vi "I2C Controller Module.vi"(11 "error in (no error)":errorcluster) -> (15 "error out":errorcluster)   [LabVIEW 2020, in "I2C Controller Lib.lvlib"]
uses:
  I2C Controller Lib.lvlib
  TypeDef/Transmission Data.ctl
  TypeDef/DVR Cluster.ctl
  Class/Transmission Mode/Parent/TX Speed.lvclass
  Class/Addressing Mode/Parent/Addressing Mode.lvclass
  Class/Devices/Parent/Devices.lvclass
  TypeDef/Path Cluster.ctl
  TypeDef/Queue Operation Mode.ctl
  TypeDef/User LV2 Mode Select.ctl
  <vilib>/Utility/config.llb/Read Key (String).vi
  Class/Transmission Mode/Child/Low Speed/SubVI/SubPanel.vi
  <vilib>/Utility/config.llb/NI_LVConfig.lvlib
  Class/Transmission Mode/Child/Low Speed/Low Speed.lvclass
panel:
  in  "Clear?":bool
  in  "Configure?":bool
  out "Warning":string caption="Warning:"
  in  "TX.Data":T1=[10, 188, 218, 14, 47, 69, 255, 107, 7, 92, 64] caption="Transmission Data" format="%.0x"
  out "RX.Data":u8[](array[numeric]) caption="Read Bytes" format="%.0x"
  out "Acknoledge?":bool caption="ACK / NACK"
  in  "Speed Mode":string(combo)="Select Device"
  in  "Transmit Data?":bool caption="Start Transmission"
  in  "Add Device?":bool caption="Add DEvice?"
  in  "Oper. Mode":string(combo)="Select Operation" caption="Operation Mode"
  in  "Address Mode":enum32{"7-bit", "10-Bit"}(radio) caption="Addressing Mode"
  in  "Log.Open?":bool
  in  "Target Address":u16=26 max=128 step=1 format="%.0x"
  in  "Device Type":string(combo)="Select Device Type"
  in  "Voltage":dbl=1.8 caption="Voltage (V)" min=1.8 max=5.0 step=1.0 format="%.2g"
  out "Digital Waveform Graph":digitaldata[](graph) caption="Graph"
  # "I2C Controller Module"
  # "Controller"
  # "Target"
  # "Transmission Parameters"
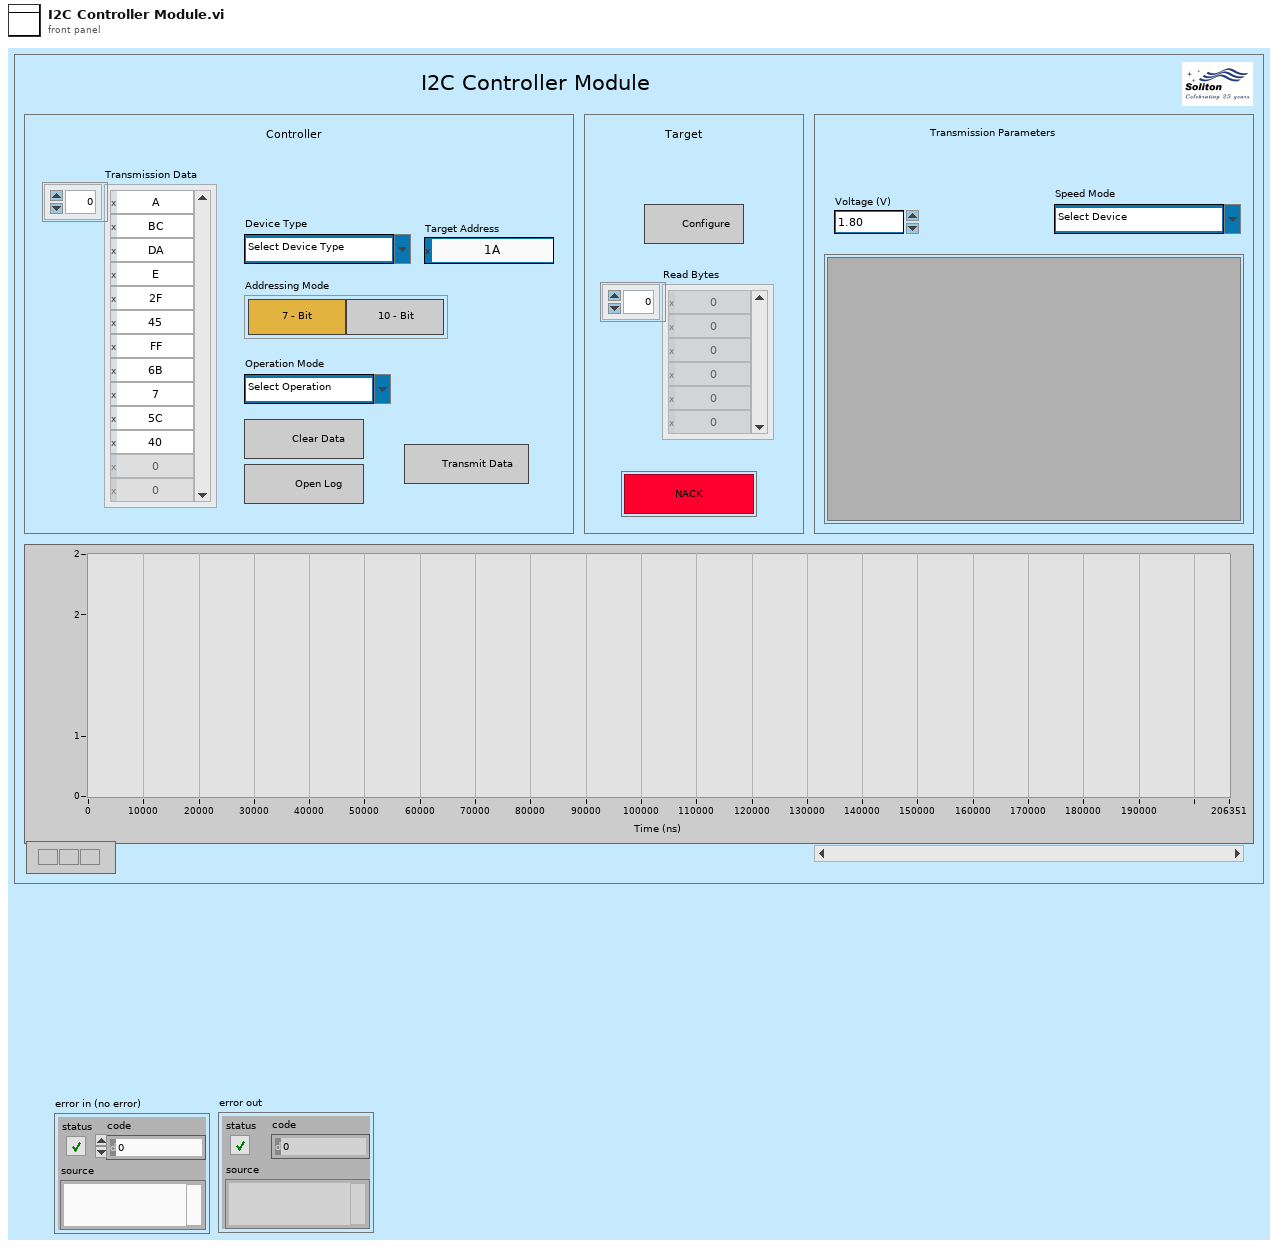
[diagram p1: front panel]
types:
  T1 = typedef "I2C Controller Lib.lvlib/Transmission Data.ctl" = u8[]
  T2 = typedef "I2C Controller Lib.lvlib/User LV2 Mode Select.ctl" = enum16{"Create", "Delete", "Stop"}
  T3 = typedef "I2C Controller Lib.lvlib/Queue Operation Mode.ctl" = enum16{"Create Q", "Enqueue", "Enqueue N", "Enstack", "Dequeue", "Flush Q", "Close Q"}
  T4 = typedef "I2C Controller Lib.lvlib/DVR Cluster.ctl" = cluster{"TX. Mode":refnum<data-value>, "Addr. Mode":refnum<data-value>, "Devices":refnum<data-value>}
  T5 = typedef "I2C Controller Lib.lvlib/Path Cluster.ctl" = cluster{"Config File":path, "TX.Mode":path, "Devices":path, "Addr. Mode":path}
  T6 = cluster{"Enable/Disable":string, "Warning":string, "Oper. Mode":string, "Speed Mode":string, "Address Mode":enum32{"7-bit", "10-Bit"}, "TX.Data":T1, "Device Type":string, "DVR":T4, "Path":T5, "Flags":cluster{"Device Type":bool, "Speed Mode":bool, "Target Address":bool, "Oper. Mode":bool}, "RX.Data":u8[], "Acknoledge?":bool, "Graph Wave":digitaldata[]}
  T7 = typedef "NI_LVConfig.lvlib/Config Data RefNum.ctl" = refnum<k1>
  T8 = enum8{"Enabled", "Disabled", "Disabled and Grayed Out"}
  T9 = cluster{"Device Type":bool, "Speed Mode":bool, "Target Address":bool, "Oper. Mode":bool}
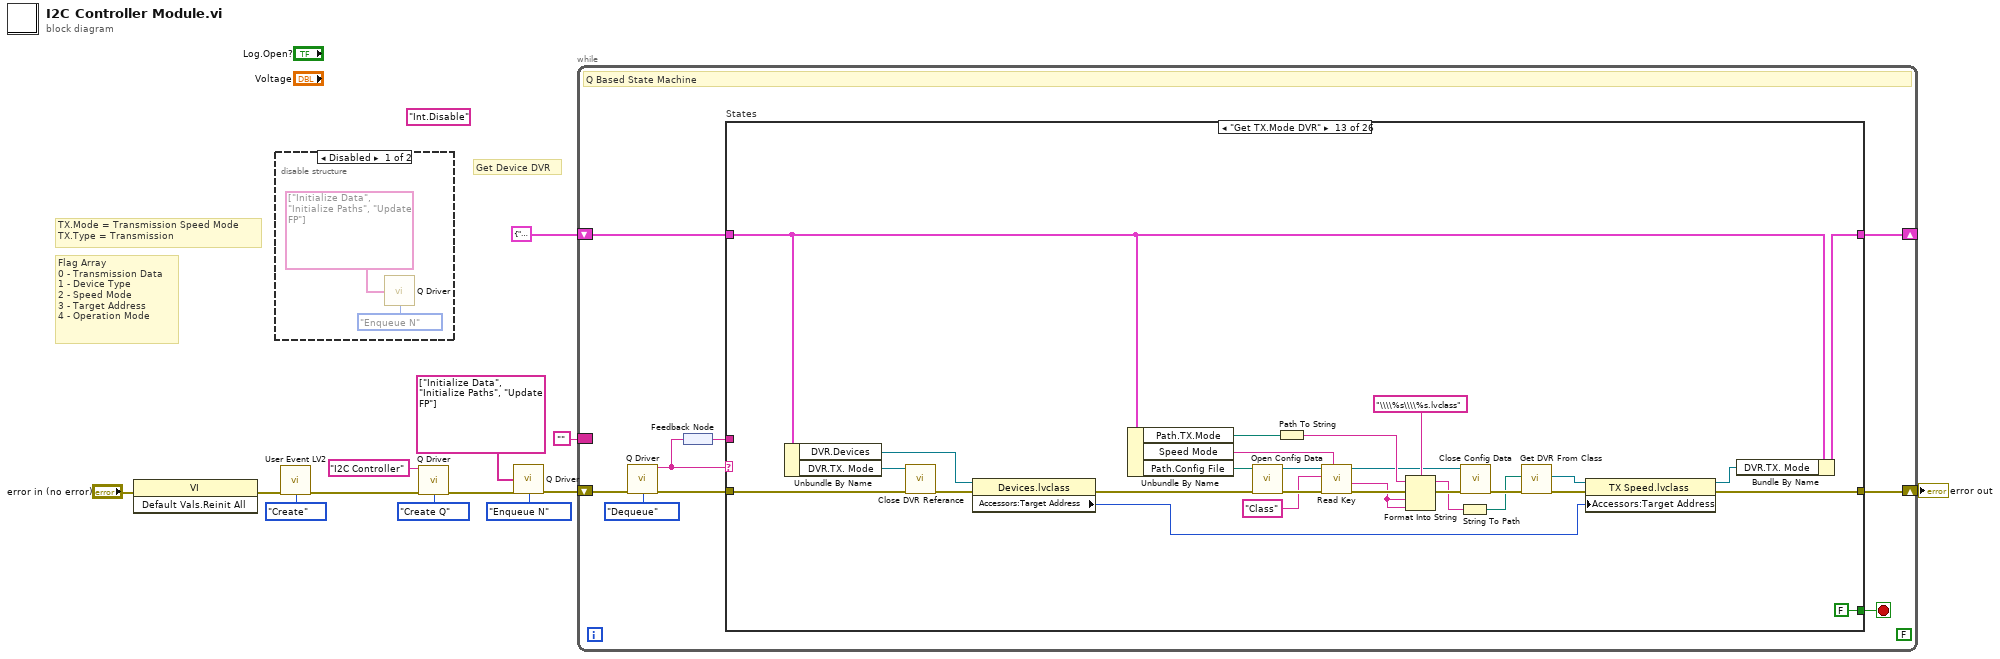
[diagram p0: block diagram]
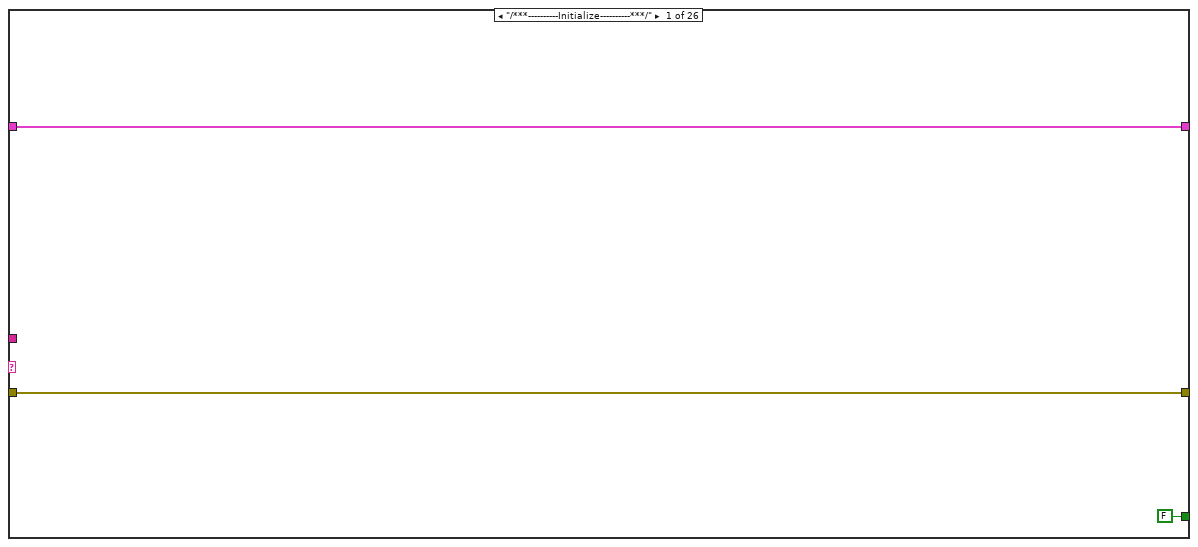
[diagram p3: hidden frame]
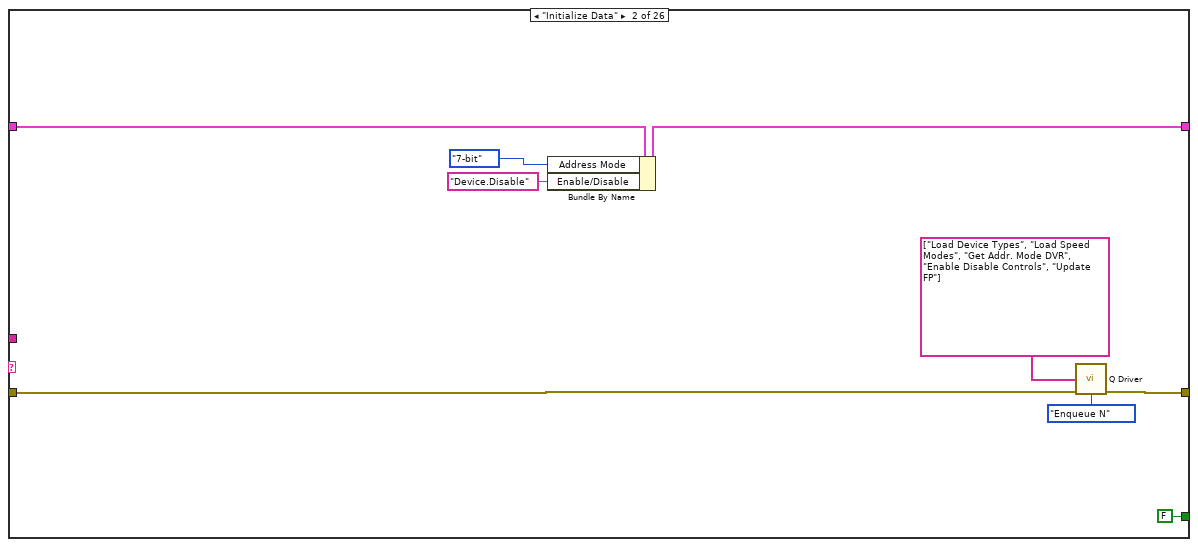
[diagram p4: hidden frame]
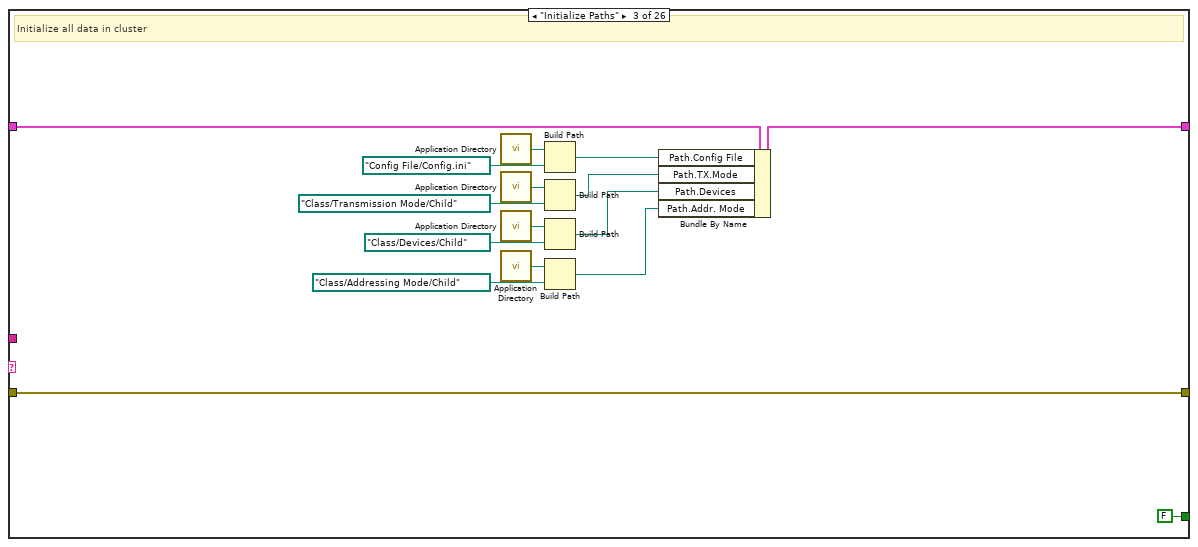
[diagram p5: hidden frame]
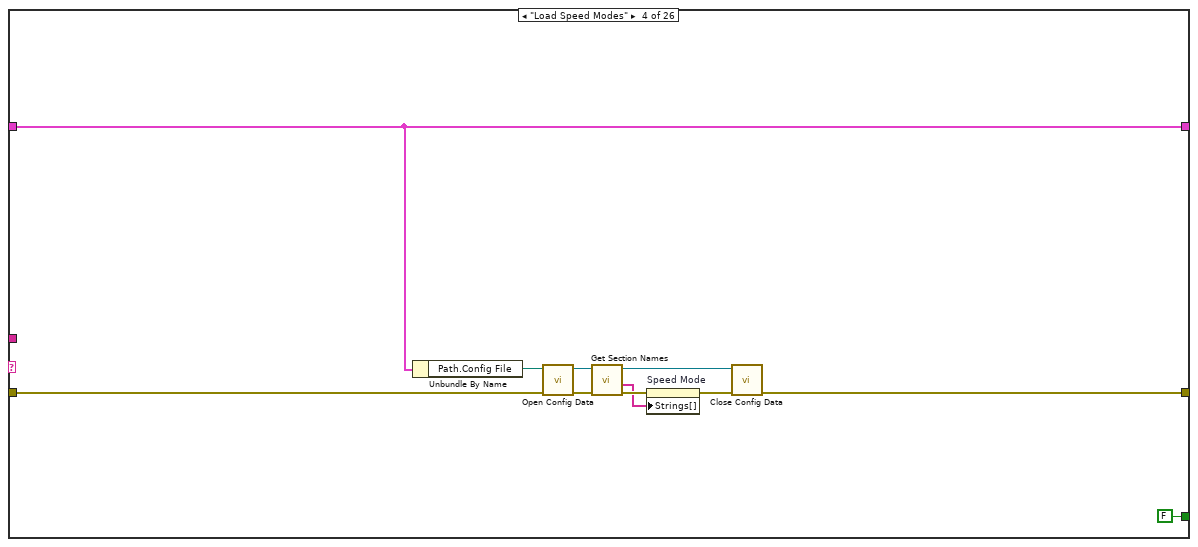
[diagram p6: hidden frame]
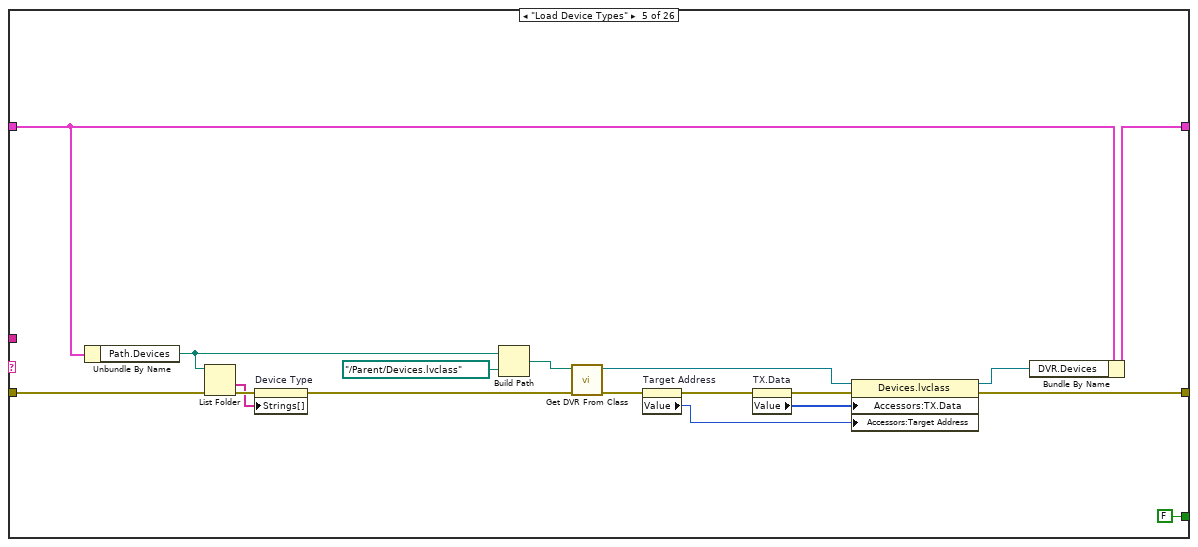
[diagram p7: hidden frame]
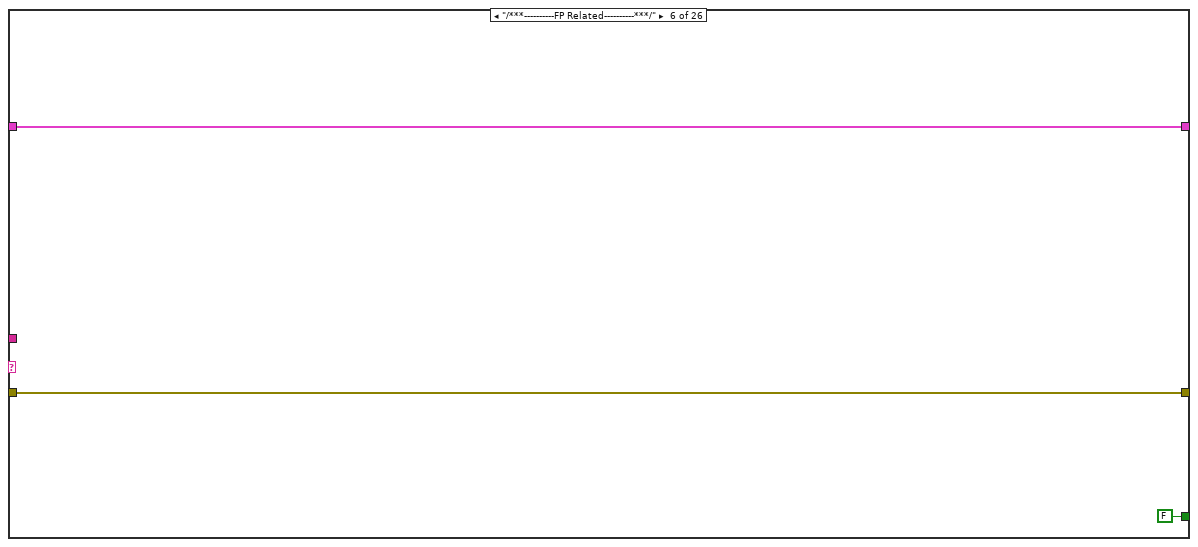
[diagram p8: hidden frame]
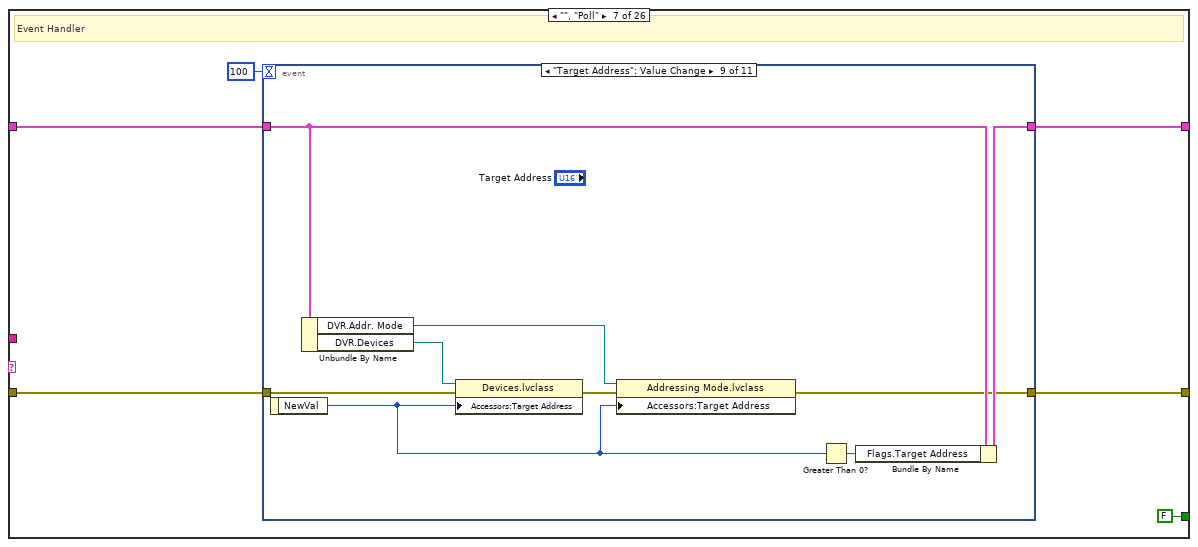
[diagram p9: hidden frame]
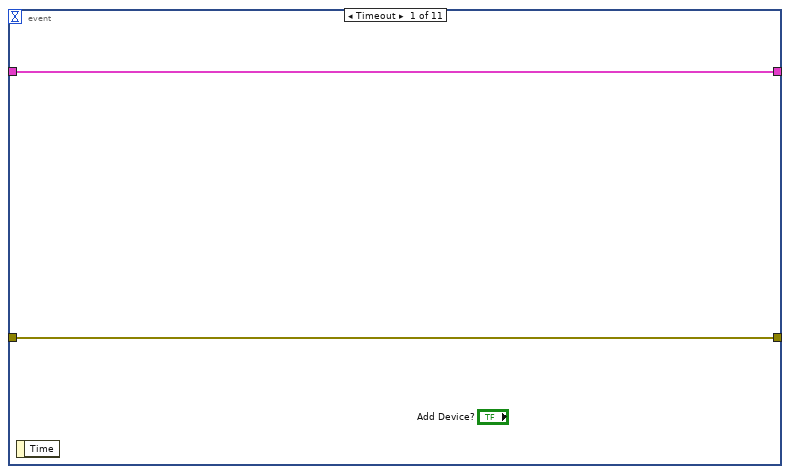
[diagram p10: hidden frame]
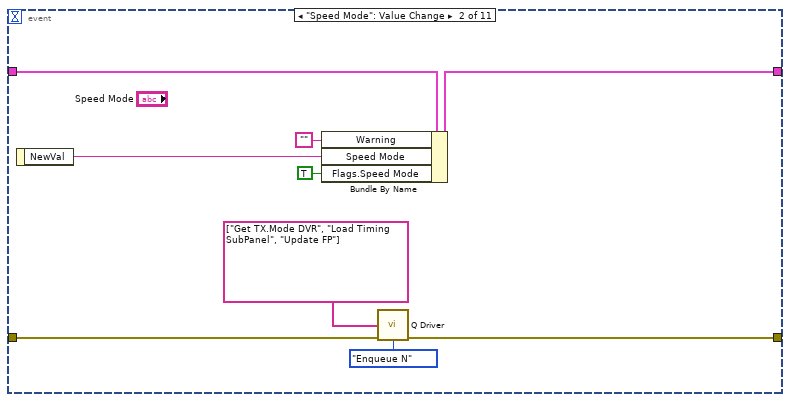
[diagram p11: hidden frame]
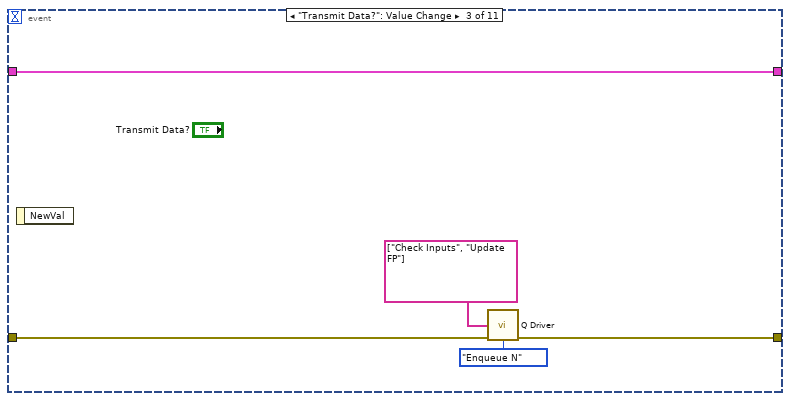
[diagram p12: hidden frame]
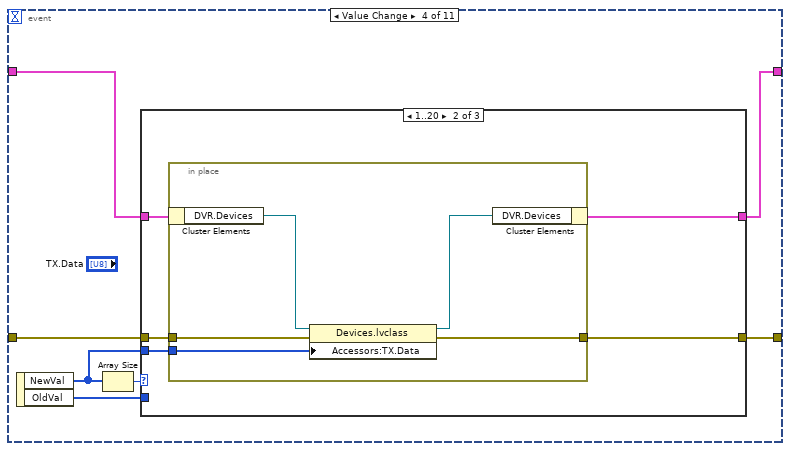
[diagram p13: hidden frame]
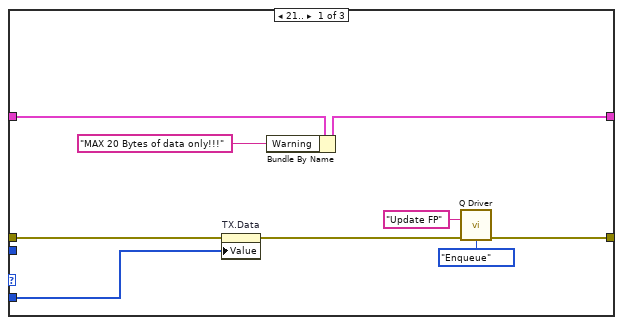
[diagram p14: hidden frame]
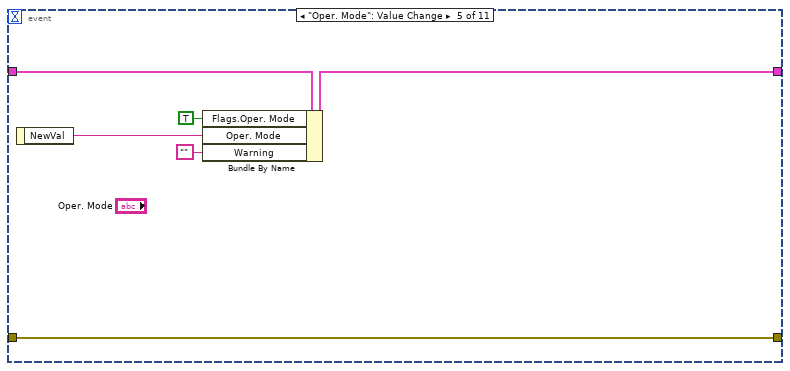
[diagram p16: hidden frame]
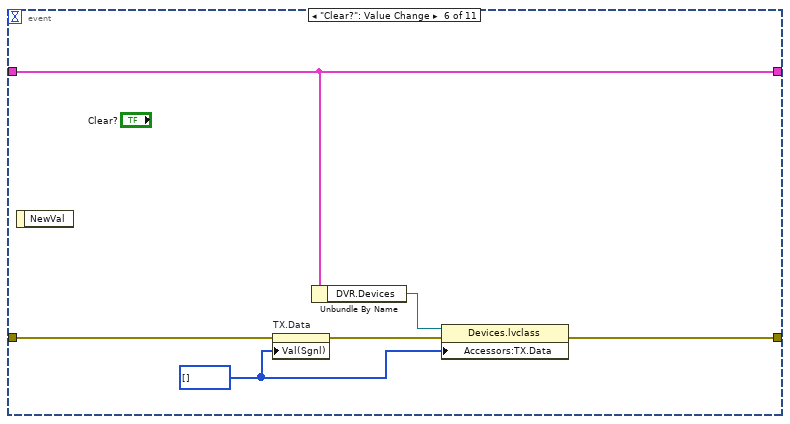
[diagram p17: hidden frame]
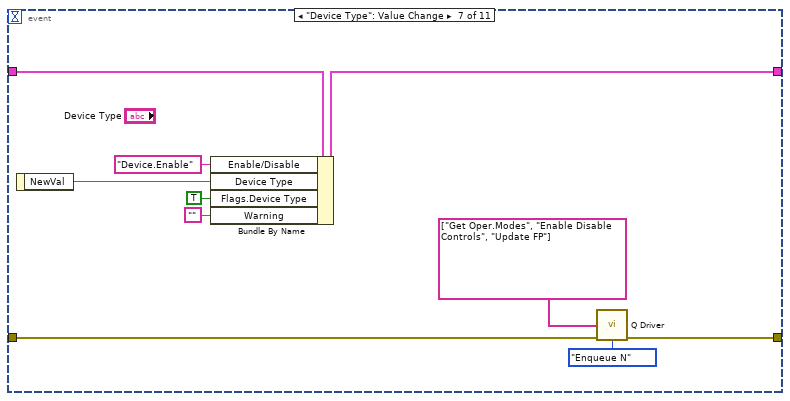
[diagram p18: hidden frame]
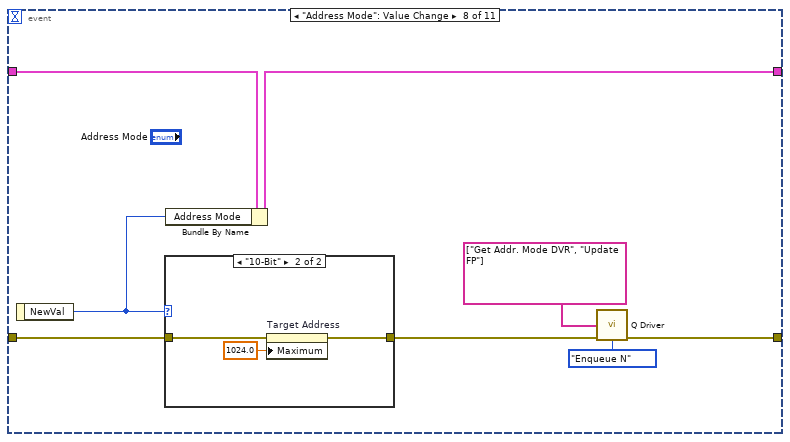
[diagram p19: hidden frame]
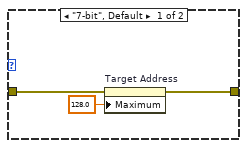
[diagram p20: hidden frame]
diagram:
  (unwired) "Int.Disable" ("Enable/Disable")
  # "Get Device DVR"
  # "Flag Array\n0 - Transmission Data\n1 - Device Type\n2 - Speed Mode\n3 - Target Address\n4 - Operation Mode"
  # "TX.Mode = Transmission Speed Mode\nTX.Type = Transmission"
  n1 = invoke class="VI" method="Default Vals.Reinit All"(error in="error in (no error)") -> (error out=w2:errorcluster)  [unwired: 2 in, 2 out]
  n2 = disable-structure shown="Disabled" {
    frame Disabled {
      n3 = call "Q Driver.vi"("States s[]"=string[] ["Initialize Data", "Initialize Paths", "Update FP"], "Q Operation"=Queue_Operation_Mode."Enqueue N") -> ()  [unwired: 12 in, 2 out]
    }
    frame Enabled {
    }
  }
  n4 = call "User Event LV2.vi"("error in (no error)"=w2, "LV2 Mode"=User_LV2_Mode_Select."Create") -> ("error out"=w1:errorcluster)  [unwired: 12 in, 1 out]
  n5 = call "Q Driver.vi"("Q Name"="I2C Controller", "error in (no error)"=w1, "Q Operation"=Queue_Operation_Mode."Create Q") -> ("error out"=w12:errorcluster)  [unwired: 11 in, 1 out]
  n6 = call "Q Driver.vi"("States s[]"=string[] ["Initialize Data", "Initialize Paths", "Update FP"], "error in (no error)"=w12, "Q Operation"=Queue_Operation_Mode."Enqueue N") -> ("error out"=w11:errorcluster)  [unwired: 11 in, 1 out]
  n7 = while {
    shift-right: [w21] -> _
    shift-left: T6 {"Enable/Disable"="", "Warning"="", "Oper. Mode"="", "Speed Mode"="", "Address Mode"=enum."7-bit", "TX.Data"=[], "Device Type"="", "DVR"={"TX. Mode"=refnum, "Addr. Mode"=refnum, "Devices"=refnum}, "Path"={"Config File"=path "", "TX.Mode"=path "", "Devices"=path "", "Addr. Mode"=path ""}, "Flags"={"Device Type"=FALSE, "Speed Mode"=FALSE, "Target Address"=TRUE, "Oper. Mode"=FALSE}, "RX.Data"=[], "Acknoledge?"=FALSE, "Graph Wave"=[]} -> [w20]
    shift-right: [w22] -> w8
    shift-left: w11 -> [w24]
    border: "" -> [_]
    stop <- w19 stop-if-true
    (unwired) FALSE
    # "Q Based State Machine"
    n8 = call "Q Driver.vi"("error in (no error)"=w24, "Q Operation"=Queue_Operation_Mode."Dequeue") -> ("State Out"=w17:string, "error out"=w23:errorcluster)  [unwired: 12 in]
    n9 = feedback-in #1(w17) -> ()
    n10 = feedback #1() -> (w16:string)
    n11 = case "States" shown="\"Get TX.Mode DVR\"" w17 {
      selector: w17 -> [_ _ _ _ _ _ _ _ _ _ _ _ _ _ _ _ _ _ _ _ _ _ _ w468 _ _]
      tunnel: w23 -> [w27 w31 w40 w62 w80 w84 w90 w207 w227 w230 w236 w250 w289 w309 w320 w326 w330 w345 w373 w426 w443 w446 w449 w470 w491 w496]
      tunnel: [w27 w30 w40 w56 w69 w84 w89 w208 w227 w230 w238 w253 w282 w309 w319 w325 w330 w337 w371 w415 w441 w446 w448 w469 w491 w494] -> w22
      tunnel: [w26 w35 w50 w54 w74 w83 w87 w206 w225 w229 w237 w254 w291 w308 w321 w324 w329 w340 w374 w413 w429 w445 w460 w481 w490 w498] -> w21
      tunnel: w20 -> [w26 w36 w51 w54 w79 w83 w86 w206 w225 w229 w244 w252 w288 w308 w321 w324 w329 w340 w376 w423 w442 w445 w460 w481 w490 w498]
      tunnel: [FALSE FALSE FALSE FALSE FALSE FALSE FALSE FALSE FALSE FALSE FALSE FALSE FALSE FALSE FALSE FALSE FALSE FALSE FALSE FALSE FALSE FALSE FALSE FALSE FALSE TRUE] -> w19
      tunnel: w16 -> [_ _ _ _ _ _ _ _ _ _ _ _ _ _ _ _ _ _ _ _ _ _ w447 _ _ _]
      frame "/***----------Initialize----------***/" {
      }
      frame "Initialize Data" {
        n12 = Bundle By Name(cluster=w36, "Address Mode"=enum32{"7-bit", "10-Bit"}."7-bit", "Enable/Disable"="Device.Disable") -> (w35:T6)
        n13 = call "Q Driver.vi"("States s[]"=string[] ["Load Device Types", "Load Speed Modes", "Get Addr. Mode DVR", "Enable Disable Controls", "Update FP"], "error in (no error)"=w31, "Q Operation"=Queue_Operation_Mode."Enqueue N") -> ("error out"=w30:errorcluster)  [unwired: 11 in, 1 out]
      }
      frame "Initialize Paths" {
        # "Initialize all data in cluster"
        n14 = call <vilib>:"Application Directory.vi"() -> ("Application Directory"=w49:path)
        n15 = call <vilib>:"Application Directory.vi"() -> ("Application Directory"=w45:path)
        n16 = call <vilib>:"Application Directory.vi"() -> ("Application Directory"=w43:path)
        n17 = call <vilib>:"Application Directory.vi"() -> ("Application Directory"=w39:path)
        n18 = Build Path(base path=w49, name or relative path=path "Config File/Config.ini" ("Config.ini")) -> (appended path=w47:path)
        n19 = Build Path(base path=w45, name or relative path=path "Class/Transmission Mode/Child" ("Config.ini")) -> (appended path=w44:path)
        n20 = Build Path(base path=w43, name or relative path=path "Class/Devices/Child" ("Config.ini")) -> (appended path=w41:path)
        n21 = Build Path(base path=w39, name or relative path=path "Class/Addressing Mode/Child" ("Config.ini")) -> (appended path=w37:path)
        n22 = Bundle By Name(cluster=w51, "Path.Config File"=w47, "Path.TX.Mode"=w44, "Path.Devices"=w41, "Path.Addr. Mode"=w37) -> (w50:T6)
      }
      frame "Load Speed Modes" {
        n23 = Unbundle By Name(w54) -> ("Path.Config File"=w53:path)
        n24 = call <vilib>:"Open Config Data.vi"("error in (no error)"=w62, "configuration file path"=w53) -> ("error out"=w61:errorcluster, "refnum"=w60:T7)  [unwired: 7 in, 1 out]
        n25 = call <vilib>:"Get Section Names.vi"("error in (no error)"=w61, "refnum"=w60) -> ("error out"=w59:errorcluster, "section names"=w58:string[], "refnum out"=w55:T7)  [unwired: 7 in]
        n26 = property on="Speed Mode" class="CmbBox"(error in=w59, "Strings[]"=w58) -> (error out=w57:errorcluster)  [unwired: 1 in, 1 out]
        n27 = call <vilib>:"Close Config Data.vi"("error in (no error)"=w57, "refnum"=w55) -> ("error out"=w56:errorcluster)  [unwired: 8 in, 1 out]
      }
      frame "Load Device Types" {
        n28 = Unbundle By Name(w79) -> ("Path.Devices"=w73:path)
        n29 = List Folder(path=w73, error in=w80) -> (folder names=w77:string[], error out=w78:errorcluster)  [unwired: 2 in, 2 out]
        n30 = property on="Device Type" class="CmbBox"(error in=w78, "Strings[]"=w77) -> (error out=w76:errorcluster)  [unwired: 1 in, 1 out]
        n31 = Build Path(base path=w73, name or relative path=path "../Parent/Devices.lvclass") -> (appended path=w72:path)
        n32 = call "Get DVR From Class.vi"("error in (no error)"=w76, "Path In"=w72) -> ("error out"=w75:errorcluster, "Devices DVR"=w68:refnum<data-value>)  [unwired: 8 in]
        n33 = property on="Target Address" class="DigNum (strict)"(error in=w75) -> (error out=w65:errorcluster, "Value"=w64:u16)  [unwired: 1 in, 1 out]
        n34 = property on="TX.Data" class="Arr (strict)"(error in=w65) -> (error out=w70:errorcluster, "Value"=w67:T1)  [unwired: 1 in, 1 out]
        n35 = property class="Devices.lvclass"(reference=w68, error in=w70, "Accessors:TX.Data"=w67, "Accessors:Target Address"=w64) -> (reference out=w66:refnum<data-value>, error out=w69:errorcluster)
        n36 = Bundle By Name(cluster=w79, "DVR.Devices"=w66) -> (w74:T6)
      }
      frame "/***----------FP Related----------***/" {
      }
      frame "", "Poll" {
        # "Event Handler"
        n37 = event shown="[8] \"Target Address\": Value Change" {
          selector: _ -> [_ _ _ _ _ _ _ _ _ _ _]
          dyn-events: _ -> [_ _ _ _ _ _ _ _ _ _ _]
          timeout: 100 -> [_ _ _ _ _ _ _ _ _ _ _]
          tunnel: w90 -> [w92 w97 w103 w113 w135 w146 w153 w163 w177 w186 w203]
          tunnel: [w92 w96 w102 w112 w135 w143 w152 w160 w172 w185 w202] -> w89
          tunnel: [w91 w100 w106 w107 w139 w144 w148 w158 w179 w183 w201] -> w87
          tunnel: w86 -> [w91 w101 w106 w111 w140 w144 w156 w164 w175 w182 w201]
          event Timeout {
            n38 = event-data() -> ()  [unwired: 1 in, 1 out]
          }
          event "Speed Mode": Value Change {
            n39 = event-data() -> ("NewVal"=w99:string)  [unwired: 1 in]
            n40 = Bundle By Name(cluster=w101, "Warning"="", "Speed Mode"=w99, "Flags.Speed Mode"=TRUE) -> (w100:T6)
            n41 = call "Q Driver.vi"("States s[]"=string[] ["Get TX.Mode DVR", "Load Timing SubPanel", "Update FP"], "error in (no error)"=w97, "Q Operation"=Queue_Operation_Mode."Enqueue N") -> ("error out"=w96:errorcluster)  [unwired: 11 in, 1 out]
          }
          event "Transmit Data?": Value Change {
            n42 = event-data() -> ()  [unwired: 1 in, 1 out]
            n43 = call "Q Driver.vi"("States s[]"=string[] ["Check Inputs", "Update FP"], "error in (no error)"=w103, "Q Operation"=Queue_Operation_Mode."Enqueue N") -> ("error out"=w102:errorcluster)  [unwired: 11 in, 1 out]
          }
          event Value Change {
            n44 = event-data() -> ("NewVal"=w110:T1, "OldVal"=w108:T1)  [unwired: 1 in]
            n45 = Array Size(array=w110) -> (size(s)=w109:i32)
            n46 = case shown="1..20" w109 {
              tunnel: w113 -> [w121 w127 w133]
              tunnel: [w119 w123 w134] -> w107
              tunnel: [w115 w126 w133] -> w112
              tunnel: w111 -> [w122 w124 w134]
              tunnel: w110 -> [_ w125 _]
              tunnel: w108 -> [w120 _ _]
              frame 21.. {
                n47 = property on="TX.Data" class="Arr (strict)"(error in=w121, "Value"=w120) -> (error out=w116:errorcluster)  [unwired: 1 in, 1 out]
                n48 = Bundle By Name(cluster=w122, "Warning"="MAX 20 Bytes of data only!!!") -> (w119:T6)
                n49 = call "Q Driver.vi"("State In"="Update FP" ("element"), "error in (no error)"=w116, "Q Operation"=Queue_Operation_Mode."Enqueue") -> ("error out"=w115:errorcluster)  [unwired: 11 in, 1 out]
              }
              frame 1..20 {
                n50 = in-place {
                  in-place-border: w127 -> [w132]
                  in-place-border: [w131] -> w126
                  in-place-border: w125 -> [w130]
                  n51 = in-place-cluster #2(w124) -> ("DVR.Devices"=w129:refnum<data-value>)
                  n52 = property class="Devices.lvclass"(reference=w129, error in=w132, "Accessors:TX.Data"=w130) -> (reference out=w128:refnum<data-value>, error out=w131:errorcluster)
                  n53 = in-place-cluster #2("DVR.Devices"=w128) -> (w123:T6)
                }
              }
              frame 0, Default {
              }
            }
          }
          event "Oper. Mode": Value Change {
            n54 = event-data() -> ("NewVal"=w137:string)  [unwired: 1 in]
            n55 = Bundle By Name(cluster=w140, "Flags.Oper. Mode"=TRUE, "Oper. Mode"=w137, "Warning"="") -> (w139:T6)
          }
          event "Clear?": Value Change {
            w141 = T1 [] ("TX.Data")
            n56 = event-data() -> ()  [unwired: 1 in, 1 out]
            n57 = property on="TX.Data" class="Arr (strict)"(error in=w146, "Val(Sgnl)"=w141) -> (error out=w145:errorcluster)  [unwired: 1 in, 1 out]
            n58 = Unbundle By Name(w144) -> ("DVR.Devices"=w142:refnum<data-value>)
            n59 = property class="Devices.lvclass"(reference=w142, error in=w145, "Accessors:TX.Data"=w141) -> (error out=w143:errorcluster)  [unwired: 1 out]
          }
          event "Device Type": Value Change {
            n60 = event-data() -> ("NewVal"=w155:string)  [unwired: 1 in]
            n61 = Bundle By Name(cluster=w156, "Enable/Disable"="Device.Enable", "Device Type"=w155, "Flags.Device Type"=TRUE, "Warning"="") -> (w148:T6)
            n62 = call "Q Driver.vi"("States s[]"=string[] ["Get Oper.Modes", "Enable Disable Controls", "Update FP"], "error in (no error)"=w153, "Q Operation"=Queue_Operation_Mode."Enqueue N") -> ("error out"=w152:errorcluster)  [unwired: 11 in, 1 out]
          }
          event "Address Mode": Value Change {
            n63 = event-data() -> ("NewVal"=w157:enum32{"7-bit", "10-Bit"})  [unwired: 1 in]
            n64 = case shown="\"10-Bit\"" w157 {
              tunnel: [w165 w169] -> w161
              tunnel: w163 -> [w166 w170]
              frame "7-bit", Default {
                n65 = property on="Target Address" class="DigNum (strict)"(error in=w166, "Maximum"=128.0 ("Data Entry Limits:Maximum")) -> (error out=w165:errorcluster)  [unwired: 1 in, 1 out]
              }
              frame "10-Bit" {
                n66 = property on="Target Address" class="DigNum (strict)"(error in=w170, "Maximum"=1024.0 ("Data Entry Limits:Maximum")) -> (error out=w169:errorcluster)  [unwired: 1 in, 1 out]
              }
            }
            n67 = Bundle By Name(cluster=w164, "Address Mode"=w157) -> (w158:T6)
            n68 = call "Q Driver.vi"("States s[]"=string[] ["Get Addr. Mode DVR", "Update FP"], "error in (no error)"=w161, "Q Operation"=Queue_Operation_Mode."Enqueue N") -> ("error out"=w160:errorcluster)  [unwired: 11 in, 1 out]
          }
          event "Target Address": Value Change {
            n69 = event-data() -> ("NewVal"=w171:u16)  [unwired: 1 in]
            n70 = Unbundle By Name(w175) -> ("DVR.Addr. Mode"=w173:refnum<data-value>, "DVR.Devices"=w174:refnum<data-value>)
            n71 = property class="Devices.lvclass"(reference=w174, error in=w177, "Accessors:Target Address"=w171) -> (error out=w176:errorcluster)  [unwired: 1 out]
            n72 = property class="Addressing Mode.lvclass"(reference=w173, error in=w176, "Accessors:Target Address"=w171) -> (error out=w172:errorcluster)  [unwired: 1 out]
            n73 = Greater Than 0?(x=w171) -> (x > 0?=w178:bool)
            n74 = Bundle By Name(cluster=w175, "Flags.Target Address"=w178) -> (w179:T6)
          }
          event "Configure?": Value Change {
            n75 = event-data() -> ()  [unwired: 1 in, 1 out]
            n76 = Unbundle By Name(w182) -> ("Flags.Device Type"=w184:bool, "Flags.Oper. Mode"=w180:bool)
            n77 = And(x=w184, y=w180) -> (x .and. y?=w181:bool)
            n78 = case shown="True" w181 {
              tunnel: w186 -> [w189 w197]
              tunnel: [w188 w196] -> w185
              tunnel: [w192 w194] -> w183
              tunnel: w182 -> [w193 w194]
              frame False {
                n79 = call "Q Driver.vi"("State In"="Update FP" ("element"), "error in (no error)"=w189, "Q Operation"=Queue_Operation_Mode."Enqueue") -> ("error out"=w188:errorcluster)  [unwired: 11 in, 1 out]
                n80 = Bundle By Name(cluster=w193, "Warning"="Select Device Type and Operation Mode") -> (w192:T6)
              }
              frame True {
                n81 = call "Q Driver.vi"("States s[]"=string[] ["Get Device DVR", "Config RX data", "Update FP"], "error in (no error)"=w197, "Q Operation"=Queue_Operation_Mode."Enqueue N") -> ("error out"=w196:errorcluster)  [unwired: 11 in, 1 out]
              }
            }
          }
          event Panel Close? {
            n82 = event-data() -> ()  [unwired: 1 in, 1 out]
            n83 = call "Q Driver.vi"("State In"="Exit" ("Q Name"), "error in (no error)"=w203, "Q Operation"=Queue_Operation_Mode."Enqueue") -> ("error out"=w202:errorcluster)  [unwired: 11 in, 1 out]
            n84 = event-data("Discard?"=TRUE) -> ()  [unwired: 1 in, 1 out]
          }
        }
      }
      frame "Enable Disable Controls" {
        # "Enable Disable required controls"
        n85 = Unbundle By Name(w206) -> ("Enable/Disable"=w205:string)
        n86 = case shown="\"Device.Disable\"" w205 {
          tunnel: [w210 w212 w216] -> w208
          tunnel: w207 -> [w210 w215 w219]
          frame Default {
          }
          frame "Device.Enable" {
            w211 = T8."Enabled" ("Disabled")
            n87 = property on="Target Address" class="DigNum (strict)"(error in=w215, "DisabledEnum"=w211) -> (error out=w214:errorcluster)  [unwired: 1 in, 1 out]
            n88 = property on="Address Mode" class="RadioBtnsControl (strict)"(error in=w214, "DisabledEnum"=w211) -> (error out=w213:errorcluster)  [unwired: 1 in, 1 out]
            n89 = property on="Oper. Mode" class="CmbBox"(error in=w213, "DisabledEnum"=w211) -> (error out=w212:errorcluster)  [unwired: 1 in, 1 out]
          }
          frame "Device.Disable" {
            w220 = T8."Disabled and Grayed Out" ("Disabled")
            n90 = property on="Target Address" class="DigNum (strict)"(error in=w219, "DisabledEnum"=w220) -> (error out=w218:errorcluster)  [unwired: 1 in, 1 out]
            n91 = property on="Address Mode" class="RadioBtnsControl (strict)"(error in=w218, "DisabledEnum"=w220) -> (error out=w217:errorcluster)  [unwired: 1 in, 1 out]
            n92 = property on="Oper. Mode" class="CmbBox"(error in=w217, "DisabledEnum"=w220) -> (error out=w216:errorcluster)  [unwired: 1 in, 1 out]
          }
        }
      }
      frame "Update FP" {
        # "Update Front Panel Controls and Indicators"
        n93 = Unbundle By Name(w225) -> ("Warning"=→"Warning":string, "RX.Data"=→"RX.Data":u8[], "Acknoledge?"=→"Acknoledge?":bool, "Graph Wave"=→"Digital Waveform Graph":digitaldata[])
      }
      frame "/***----------DVR Functions----------***/" {
      }
      frame "Get Addr. Mode DVR" {
        n94 = Unbundle By Name(w244) -> ("Path.Addr. Mode"=w242:path, "Address Mode"=w231:enum32{"7-bit", "10-Bit"}, "DVR.Addr. Mode"=w234:refnum<data-value>)
        n95 = call "Close DVR Referance.vi"("error in (no error)"=w236, "Addr. Mode DVR"=w234) -> ("error out"=w235:errorcluster)  [unwired: 9 in]
        n96 = Path To String(path=w242) -> (string=w243:string)
        n97 = Format Into String(format string="\\\\%s\\\\%s.lvclass", initial string=w243, error in=w235, w231, w231) -> (resulting string=w240:string, error out=w239:errorcluster)
        n98 = String To Path(string=w240) -> (path=w232:path)
        n99 = call "Get DVR From Class.vi"("error in (no error)"=w239, "Path In"=w232) -> ("error out"=w238:errorcluster, "Addr. Mode DVR"=w233:refnum<data-value>)  [unwired: 8 in]
        n100 = Bundle By Name(cluster=w244, "DVR.Addr. Mode"=w233) -> (w237:T6)
      }
      frame "Get Device DVR" {
        n101 = Unbundle By Name(w252) -> ("Device Type"=w248:string, "DVR.Devices"=w251:refnum<data-value>)
        n102 = call "Get Class From DVR.vi"("error in (no error)"=w250, "Devices DVR IN"=w251) -> ("error out"=w249:errorcluster, "Class name"=w246:string)  [unwired: 7 in, 1 out]
        n103 = Equal?(x=w248, y=w246) -> (x = y?=w247:bool)
        n104 = case shown="False" w247 {
          tunnel: w249 -> [w276 w278]
          tunnel: w252 -> [w275 w277]
          tunnel: [w270 w277] -> w254
          tunnel: [w266 w278] -> w253
          frame False {
            n105 = Unbundle By Name(w275) -> ("Path.Devices"=w267:path, "Device Type"=w258:string, "Oper. Mode"=w257:string, "DVR.Devices"=w264:refnum<data-value>)
            n106 = property class="Devices.lvclass"(reference=w264, error in=w276) -> (reference out=w260:refnum<data-value>, error out=w262:errorcluster, "Accessors:TX.Data"=w263:T1, "Accessors:RX.Data"=w256:u8[])
            n107 = call "Close DVR Referance.vi"("error in (no error)"=w262, "Devices DVR"=w260) -> ("error out"=w261:errorcluster)  [unwired: 9 in]
            n108 = Path To String(path=w267) -> (string=w274:string)
            n109 = Format Into String(format string="\\\\%s\\\\Child\\\\%s\\\\%s.lvclass", initial string=w274, error in=w261, w258, w257, w257) -> (resulting string=w271:string, error out=w272:errorcluster)
            n110 = String To Path(string=w271) -> (path=w268:path)
            n111 = call "Get DVR From Class.vi"("error in (no error)"=w272, "Path In"=w268) -> ("error out"=w269:errorcluster, "Devices DVR"=w265:refnum<data-value>)  [unwired: 8 in]
            n112 = property class="Devices.lvclass"(reference=w265, error in=w269, "Accessors:TX.Data"=w263, "Accessors:RX.Data"=w256) -> (reference out=w259:refnum<data-value>, error out=w266:errorcluster)
            n113 = Bundle By Name(cluster=w275, "DVR.Devices"=w259) -> (w270:T6)
          }
          frame True {
          }
        }
      }
      frame "Get TX.Mode DVR" {
        n114 = Unbundle By Name(w288) -> ("DVR.Devices"=w283:refnum<data-value>, "DVR.TX. Mode"=w286:refnum<data-value>)
        n115 = call "Close DVR Referance.vi"("error in (no error)"=w289, "DVR IN"=w286) -> ("error out"=w287:errorcluster)  [unwired: 9 in]
        n116 = property class="Devices.lvclass"(reference=w283, error in=w287) -> (error out=w284:errorcluster, "Accessors:Target Address"=w280:u16)  [unwired: 1 out]
        n117 = Unbundle By Name(w288) -> ("Path.TX.Mode"=w300:path, "Speed Mode"=w302:string, "Path.Config File"=w303:path)
        n118 = call <vilib>:"Open Config Data.vi"("error in (no error)"=w284, "configuration file path"=w303) -> ("error out"=w306:errorcluster, "refnum"=w304:T7)  [unwired: 7 in, 1 out]
        n119 = Path To String(path=w300) -> (string=w299:string)
        n120 = call-poly <vilib>:"Read Key.vi"("section"=w302, "error in (no error)"=w306, "key"="Class", "refnum"=w304) -> ("error out"=w305:errorcluster, "value"=w285:string, "refnum out"=w296:T7)  [unwired: 4 in, 1 out]
        n121 = Format Into String(format string="\\\\%s\\\\%s.lvclass", initial string=w299, error in=w305, w285, w285) -> (resulting string=w293:string, error out=w297:errorcluster)
        n122 = String To Path(string=w293) -> (path=w292:path)
        n123 = call <vilib>:"Close Config Data.vi"("error in (no error)"=w297, "refnum"=w296) -> ("error out"=w295:errorcluster)  [unwired: 8 in, 1 out]
        n124 = call "Get DVR From Class.vi"("error in (no error)"=w295, "Path In"=w292) -> ("error out"=w294:errorcluster, "Class DVR"=w281:refnum<data-value>)  [unwired: 7 in, 1 out]
        n125 = property class="TX Speed.lvclass"(reference=w281, error in=w294, "Accessors:Target Address"=w280) -> (reference out=w279:refnum<data-value>, error out=w282:errorcluster)
        n126 = Bundle By Name(cluster=w288, "DVR.TX. Mode"=w279) -> (w291:T6)
      }
      frame "/***----------Device Type Functions----------***/" {
      }
      frame "Get Oper.Modes" {
        n127 = Unbundle By Name(w321) -> ("Path.Devices"=w315:path, "Device Type"=w313:string)
        n128 = Path To String(path=w315) -> (string=w314:string)
        n129 = Format Into String(format string="\\\\%s\\\\Child", initial string=w314, error in=w320, w313) -> (resulting string=w311:string, error out=w316:errorcluster)
        n130 = String To Path(string=w311) -> (path=w310:path)
        n131 = List Folder(path=w310, error in=w316) -> (folder names=w317:string[], error out=w318:errorcluster)  [unwired: 2 in, 2 out]
        n132 = property on="Oper. Mode" class="CmbBox"(error in=w318, "Strings[]"=w317) -> (error out=w319:errorcluster)  [unwired: 1 in, 1 out]
      }
      frame "Config RX data" {
        n133 = Unbundle By Name(w324) -> ("DVR.Devices"=w323:refnum<data-value>)
        n134 = call "SubVI Config API.vi"("error in (no error)"=w326, "Devices DVR In"=w323) -> ("error out"=w325:errorcluster)  [unwired: 8 in, 1 out]
      }
      frame "/***----------Program Functionality----------***/" {
      }
      frame "Load Timing SubPanel" {
        n135 = call "User Event LV2.vi"("error in (no error)"=w345, "LV2 Mode"=User_LV2_Mode_Select."Stop") -> ("error out"=w338:errorcluster)  [unwired: 12 in, 1 out]
        n136 = Unbundle By Name(w340) -> ("Path.TX.Mode"=w354:path, "Speed Mode"=w356:string, "Path.Config File"=w357:path)
        n137 = call <vilib>:"Open Config Data.vi"("error in (no error)"=w338, "configuration file path"=w357) -> ("error out"=w360:errorcluster, "refnum"=w358:T7)  [unwired: 7 in, 1 out]
        n138 = Path To String(path=w354) -> (string=w353:string)
        n139 = call-poly <vilib>:"Read Key.vi"("section"=w356, "error in (no error)"=w360, "key"="Class", "refnum"=w358) -> ("error out"=w359:errorcluster, "value"=w351:string, "refnum out"=w346:T7)  [unwired: 4 in, 1 out]
        n140 = Unbundle By Name(w340) -> ("DVR.TX. Mode"=w339:refnum<data-value>, "Speed Mode"=w331:string)
        n141 = Format Into String(format string="\\\\%s\\\\SubVI\\\\SubPanel.vi", initial string=w353, error in=w359, w351) -> (resulting string=w349:string, error out=w348:errorcluster)
        n142 = String To Path(string=w349) -> (path=w342:path)
        n143 = vi-ref "Low Speed.lvclass:SubPanel.vi"() -> (w334:refnum<vi>)
        n144 = Open VI Reference(type specifier VI Refnum (for type only)=w334, vi path=w342, options=256, error in (no error)=w348) -> (vi reference=w333:refnum<vi>, error out=w343:errorcluster)  [unwired: 2 in]
        n145 = call-by-ref "Start Asynchronous Call"(reference=w333, error in=w343, "DVR In"=w339, "Speed Mode"=w331) -> (error out=w336:errorcluster)  [unwired: 12 in, 3 out]
        n146 = Open VI Reference(vi path=w342, error in (no error)=w336) -> (vi reference=w332:refnum<vi>, error out=w341:errorcluster)  [unwired: 4 in]
        n147 = invoke on="Timing Panel" class="SubPnl" method="Insert VI"(error in=w341, "VI Ref"=w332) -> (error out=w350:errorcluster)  [unwired: 2 in, 3 out]
        n148 = Close Reference(reference=w332, error in (no error)=w350) -> (error out=w347:errorcluster)
        n149 = call <vilib>:"Close Config Data.vi"("error in (no error)"=w347, "refnum"=w346) -> ("error out"=w337:errorcluster)  [unwired: 8 in, 1 out]
      }
      frame "Check Inputs" {
        n150 = Unbundle By Name(w376) -> ("Flags"=w375:T9, "DVR.Devices"=w367:refnum<data-value>)
        n151 = property class="Devices.lvclass"(reference=w367, error in=w373) -> (error out=w368:errorcluster, "Accessors:TX.Data"=w366:T1, "Accessors:RX.Data"=w365:u8[])  [unwired: 1 out]
        n152 = Cluster To Array(cluster=w375) -> (array=w370:bool[])
        n153 = And Array Elements(Boolean array=w370) -> (logical AND=w372:bool)
        n154 = Empty Array?(array=w366) -> (empty?=w363:bool)
        n155 = Empty Array?(array=w365) -> (empty?=w364:bool)
        n156 = And(x=w363, y=w364) -> (x .and. y?=w362:bool)
        n157 = case shown="True" w372 {
          tunnel: [w380 w403] -> w371
          tunnel: w368 -> [w380 w404]
          tunnel: w370 -> [w379 _]
          tunnel: [w378 w402] -> w369
          tunnel: w362 -> [_ w401]
          frame False {
            n158 = for {
              tunnel: w379 -> [w383] mode=indexing
              tunnel: [w382] -> w378
              i -> [w384]
              stop <- w381 stop-if-true
              n159 = Not(x=w383) -> (.not. x?=w381:bool)
              n160 = case shown="0, Default" w384 {
                tunnel: [w387 w391 w395 w399] -> w382
                tunnel: w383 -> [w388 w392 w396 w400]
                frame 0, Default {
                  n161 = Select(t="", s=w388, f="Select Device Type") -> (s? t:f=w387:string)
                }
                frame 1 {
                  n162 = Select(t="", s=w392, f="Select Speed Mode") -> (s? t:f=w391:string)
                }
                frame 2 {
                  n163 = Select(t="", s=w396, f="Target Address Invalid") -> (s? t:f=w395:string)
                }
                frame 3 {
                  n164 = Select(t="", s=w400, f="Select Operation Mode") -> (s? t:f=w399:string)
                }
              }
            }
          }
          frame True {
            n165 = case shown="False" w401 {
              tunnel: w404 -> [w407 w410]
              tunnel: [w406 w410] -> w403
              tunnel: ["Transmission Started" "Both TX and RX Data is empty!!!"] -> w402
              frame False {
                # "All inputs present - Transmit data"
                n166 = call "Q Driver.vi"("States s[]"=string[] ["Get Device DVR", "Transmit Data", "Create Waveform", "Update FP"], "error in (no error)"=w407, "Q Operation"=Queue_Operation_Mode."Enqueue N") -> ("error out"=w406:errorcluster)  [unwired: 11 in, 1 out]
              }
              frame True {
                # "Both TX and RX Data is empty!!!"
              }
            }
          }
        }
        n167 = Bundle By Name(cluster=w376, "Warning"=w369) -> (w374:T6)
      }
      frame "Transmit Data" {
        n168 = Unbundle By Name(w423) -> ("DVR.Devices"=w420:refnum<data-value>)
        n169 = Unbundle By Name(w423) -> ("DVR.Addr. Mode"=w422:refnum<data-value>, "DVR.TX. Mode"=w421:refnum<data-value>)
        n170 = property class="Devices.lvclass"(reference=w420, error in=w426, "Accessors:Addr. Mode"=w422, "Accessors:TX. Mode"=w421) -> (reference out=w419:refnum<data-value>, error out=w417:errorcluster)
        n171 = call "Check Read_Write API.vi"("error in (no error)"=w417, "Devices DVR In"=w419) -> ("error out"=w416:errorcluster, "Devices DVR Out"=w418:refnum<data-value>)  [unwired: 8 in]
        n172 = call "Calculate I2C API.vi"("error in (no error)"=w416, "Devices DVR In"=w418) -> ("error out"=w424:errorcluster, "Devices DVR Out"=w414:refnum<data-value>)  [unwired: 8 in]
        n173 = property class="Devices.lvclass"(reference=w414, error in=w424) -> (error out=w415:errorcluster, "Accessors:RX.Data"=w412:u8[])  [unwired: 1 out]
        n174 = Bundle By Name(cluster=w423, "RX.Data"=w412) -> (w413:T6)
      }
      frame "Create Waveform" {
        n175 = Unbundle By Name(w442) -> ("DVR.TX. Mode"=w440:refnum<data-value>)
        n176 = property class="TX Speed.lvclass"(reference=w440, error in=w443) -> (error out=w441:errorcluster, "Accessors:SDA Data"=w432:u8[], "Accessors:SDA Transition"=w439:u32[], "Accessors:SCL Data"=w434:u8[], "Accessors:SCL Transition"=w433:u32[])  [unwired: 1 out]
        n177 = Build Array(w434) -> (w435:u8[][])
        n178 = Build Array(w432) -> (w438:u8[][])
        n179 = Transpose 2D Array(2D array=w438) -> (transposed array=w437:u8[][])
        n180 = Transpose 2D Array(2D array=w435) -> (transposed array=w436:u8[][])
        n181 = Bundle By Name("data"=w437, "transitions"=w439) -> (w431:digitaldata)  [unwired: 1 in]
        n182 = Bundle By Name("data"=w436, "transitions"=w433) -> (w430:digitaldata)  [unwired: 1 in]
        n183 = Build Array(w431, w430) -> (w428:digitaldata[])
        n184 = Bundle By Name(cluster=w442, "Graph Wave"=w428) -> (w429:T6)
      }
      frame "/***----------Error----------***/" {
      }
      frame "Error" {
        # "Handle Errors"
        n185 = Unbundle By Name(w449) -> ("code"=w456:i32, "source"=w455:string)
        n186 = call <vilib>:"Clear Errors.vi"("error in (no error)"=w449, "specific error code to clear (0: all)"=w456) -> ("error out"=w458:errorcluster)  [unwired: 4 in, 1 out]
        n187 = Format Into String(format string="PROGRAM ERROR\nState \"%s\".\nError Code: %d\nError Source: %s\n\nDo you wish to continue?", error in=w458, w447, w456, w455) -> (resulting string=w454:string, error out=w450:errorcluster)  [unwired: 1 in]
        n188 = Two Button Dialog(message=w454, 1:"Exit" ("F button name (\"Cancel\")"), 2:"Continue" ("T button name (\"OK\")")) -> (T button?=w451:bool)
        n189 = case "Continue?" shown="True" w451 {
          tunnel: w450 -> [w466 w467]
          tunnel: [w463 w467] -> w448
          frame False {
            # "Exit"
            n190 = call "Q Driver.vi"("error in (no error)"=w466, "Q Operation"=Queue_Operation_Mode."Flush Q") -> ("error out"=w464:errorcluster)  [unwired: 12 in, 1 out]
            n191 = call "Q Driver.vi"("State In"="Exit" ("States[]"), "error in (no error)"=w464, "Q Operation"=Queue_Operation_Mode."Enqueue") -> ("error out"=w463:errorcluster)  [unwired: 11 in, 1 out]
          }
          frame True {
            # "Continue"
          }
        }
      }
      frame "Developer Error", Default {
        # "Handle Errors"
        n192 = Unbundle By Name(w470) -> ("code"=w477:i32, "source"=w476:string)
        n193 = call <vilib>:"Clear Errors.vi"("error in (no error)"=w470, "specific error code to clear (0: all)"=w477) -> ("error out"=w479:errorcluster)  [unwired: 4 in, 1 out]
        n194 = Format Into String(format string="DEVELOPER ERROR\nState \"%s\" not found!!\nError Code: %d\nError Source: %s\n\nDo you wish to continue?", error in=w479, w468, w477, w476) -> (resulting string=w475:string, error out=w471:errorcluster)  [unwired: 1 in]
        n195 = Two Button Dialog(message=w475, 1:"Exit" ("F button name (\"Cancel\")"), 2:"Continue" ("T button name (\"OK\")")) -> (T button?=w472:bool)
        n196 = case "Continue?" shown="False" w472 {
          tunnel: w471 -> [w487 w488]
          tunnel: [w484 w488] -> w469
          frame False {
            # "Exit"
            n197 = call "Q Driver.vi"("error in (no error)"=w487, "Q Operation"=Queue_Operation_Mode."Flush Q") -> ("error out"=w485:errorcluster)  [unwired: 12 in, 1 out]
            n198 = call "Q Driver.vi"("State In"="Exit" ("States[]"), "error in (no error)"=w485, "Q Operation"=Queue_Operation_Mode."Enqueue") -> ("error out"=w484:errorcluster)  [unwired: 11 in, 1 out]
          }
          frame True {
            # "Continue"
          }
        }
      }
      frame "/***----------Exit----------***/" {
      }
      frame "Exit" {
        # "Exit the State Machine"
        n199 = call "Q Driver.vi"("error in (no error)"=w496, "Q Operation"=Queue_Operation_Mode."Flush Q") -> ("error out"=w495:errorcluster)  [unwired: 12 in, 1 out]
        n200 = call "Q Driver.vi"("error in (no error)"=w495, "Q Operation"=Queue_Operation_Mode."Close Q") -> ("error out"=w494:errorcluster)  [unwired: 12 in, 1 out]
      }
    }
  }
  "error out" <- w8
